vi "WiFi Config.vi"() -> (0 "IP Address":string)   [LabVIEW 2015]
uses:
  <vilib>/LAVA/UI Tools/Engine/Move Speed__lava_lib_ui_tools.ctl
  <vilib>/Utility/miscctls.llb/LVPositionTypeDef.ctl
  Utilities/G1.vi
  <vilib>/Platform/browser.llb/Open URL in Default Browser (string).vi
  <vilib>/MakerHub/Toolbox/LMH-Toolbox.lvlib
panel:
  in  "Overall Help 2":bool
  out "Help 2":string
  out "Tab Control":T1(tab)
  in  "INIT CANCEL":bool
  in  "INIT FRONT":bool
  in  "CON":enum32{"Y", "N"}(radio)
  in  "CON CANCEL":bool
  in  "CON FRONT":bool
  in  "CON BK":bool
  in  "H2 CANCEL":bool
  in  "H1 FRONT":bool
  in  "H1 BK":bool
  in  "H1 CANCEL":bool
  in  "H2 FRONT":bool
  in  "H2 BK":bool
  in  "CONFIG BI WIFI":bool
  in  "CONFIG CUS WIFI":bool
  out "Built-in WiFi":string="172.16.0.1"
  out "USB":string="172.22.11.2"
  in  "H3 CANCEL":bool
  in  "H3 FRONT":bool
  in  "H3 BK":bool
  in  "H4 CANCEL":bool
  in  "H4 FRONT":bool
  in  "H4 BK":bool
  in  "TELL CANCEL":bool
  in  "TELL FRONT":bool
  in  "TELL BK":bool
  in  "TELL CUSTOM IP":string caption="Please enter the IP address"
  in  "Select one":u16(ring)=1 items=["USB", "Built-in WiFi", "Custom WiFi"]
  in  "Finish":bool
  # "Communication Wizard"
  # "Hi! This is your first\nstep in starting the\nrobot. Go ahead!!"
  # "myRIO Connected??\nHave you connected the myRIO\nto your system yet??"
  # "Conecting myRIO: Step 1\nFirst power up myRIO. Wait\nfor a couple of minutes.\nConnect the myRIO via USB or WiFi."
  # "These two should light\nup. \"STATUS\" will turn\noff soon"
  # "Step 2\nOpen the project explorer. Right-click\non myRIO and open properties."
  # "ILLUSTRATION ONLY"
  # "Step 3\nEnter the IP Adddress of myRIO. A\ntable of IP addresses is given below.\nOnce done, click OK."
  # "ILLUSTRATION ONLY"
  # "If you wish to copy the addresses,\ndo it from below"
  # "Step 4\nRight-click on myRIO and\nclick on connect. If you\nget a prompt like the one\nshown in \"Fig 1\" click OK\nor Apply."
  # "ILLUSTRATION ONLY"
  # "Fig 1"
  # "What have you done??\nPlease tell us how have you\nconnected to myRIO. Choose\none option below"
  # "Done!!\nYou are done with connecting with\nmyRIO. Click finish to proceed on to\nthe settings for the robot"
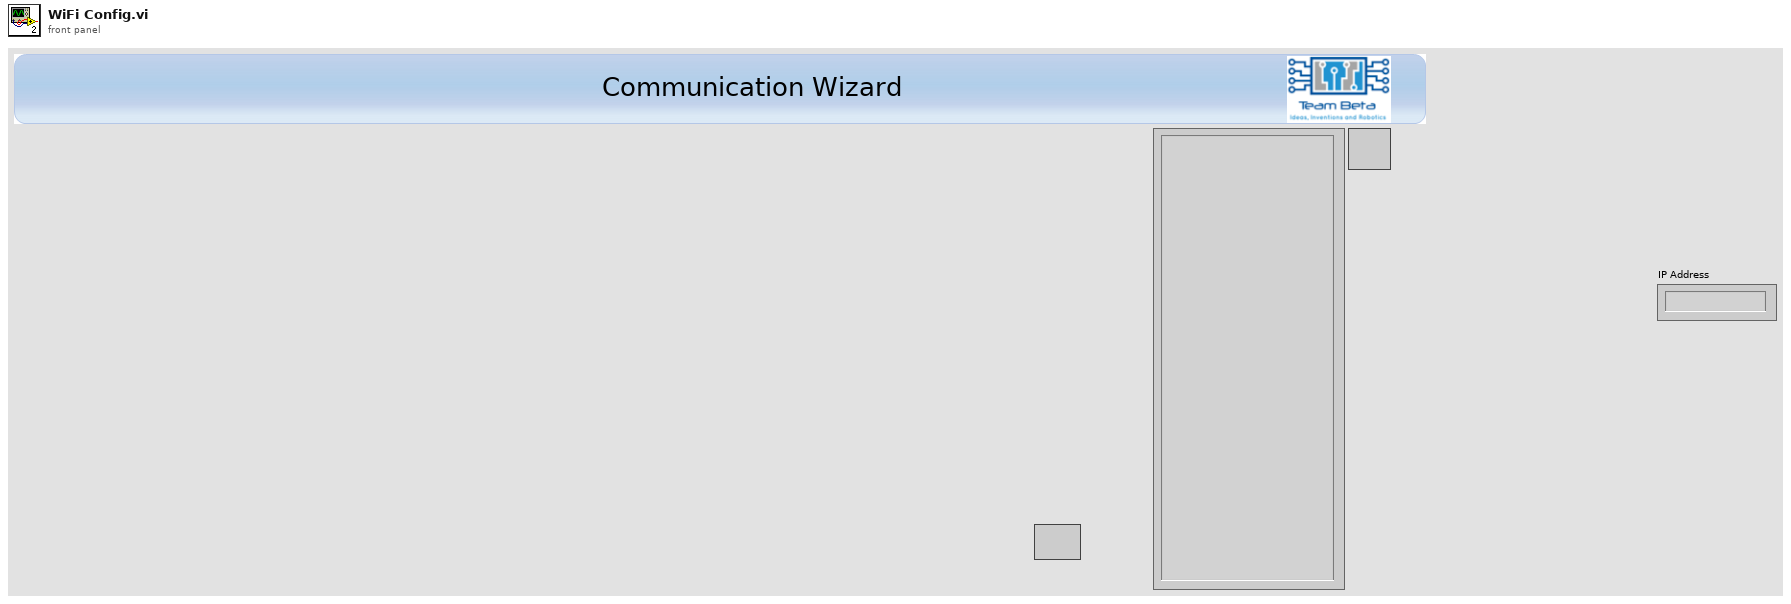
[diagram p1: front panel]
types:
  T1 = enum32{"Init", "myRIO connected?", "H1", "H2", "H3", "H4", "Tell", "Done"}
  T2 = typedef "LVPositionTypeDef.ctl" = cluster{"Left":i32, "Top":i32}
  T3 = typedef "Move Speed__lava_lib_ui_tools.ctl" = enum16{"Normal", "Fast", "Slow", "Instantaneous"}
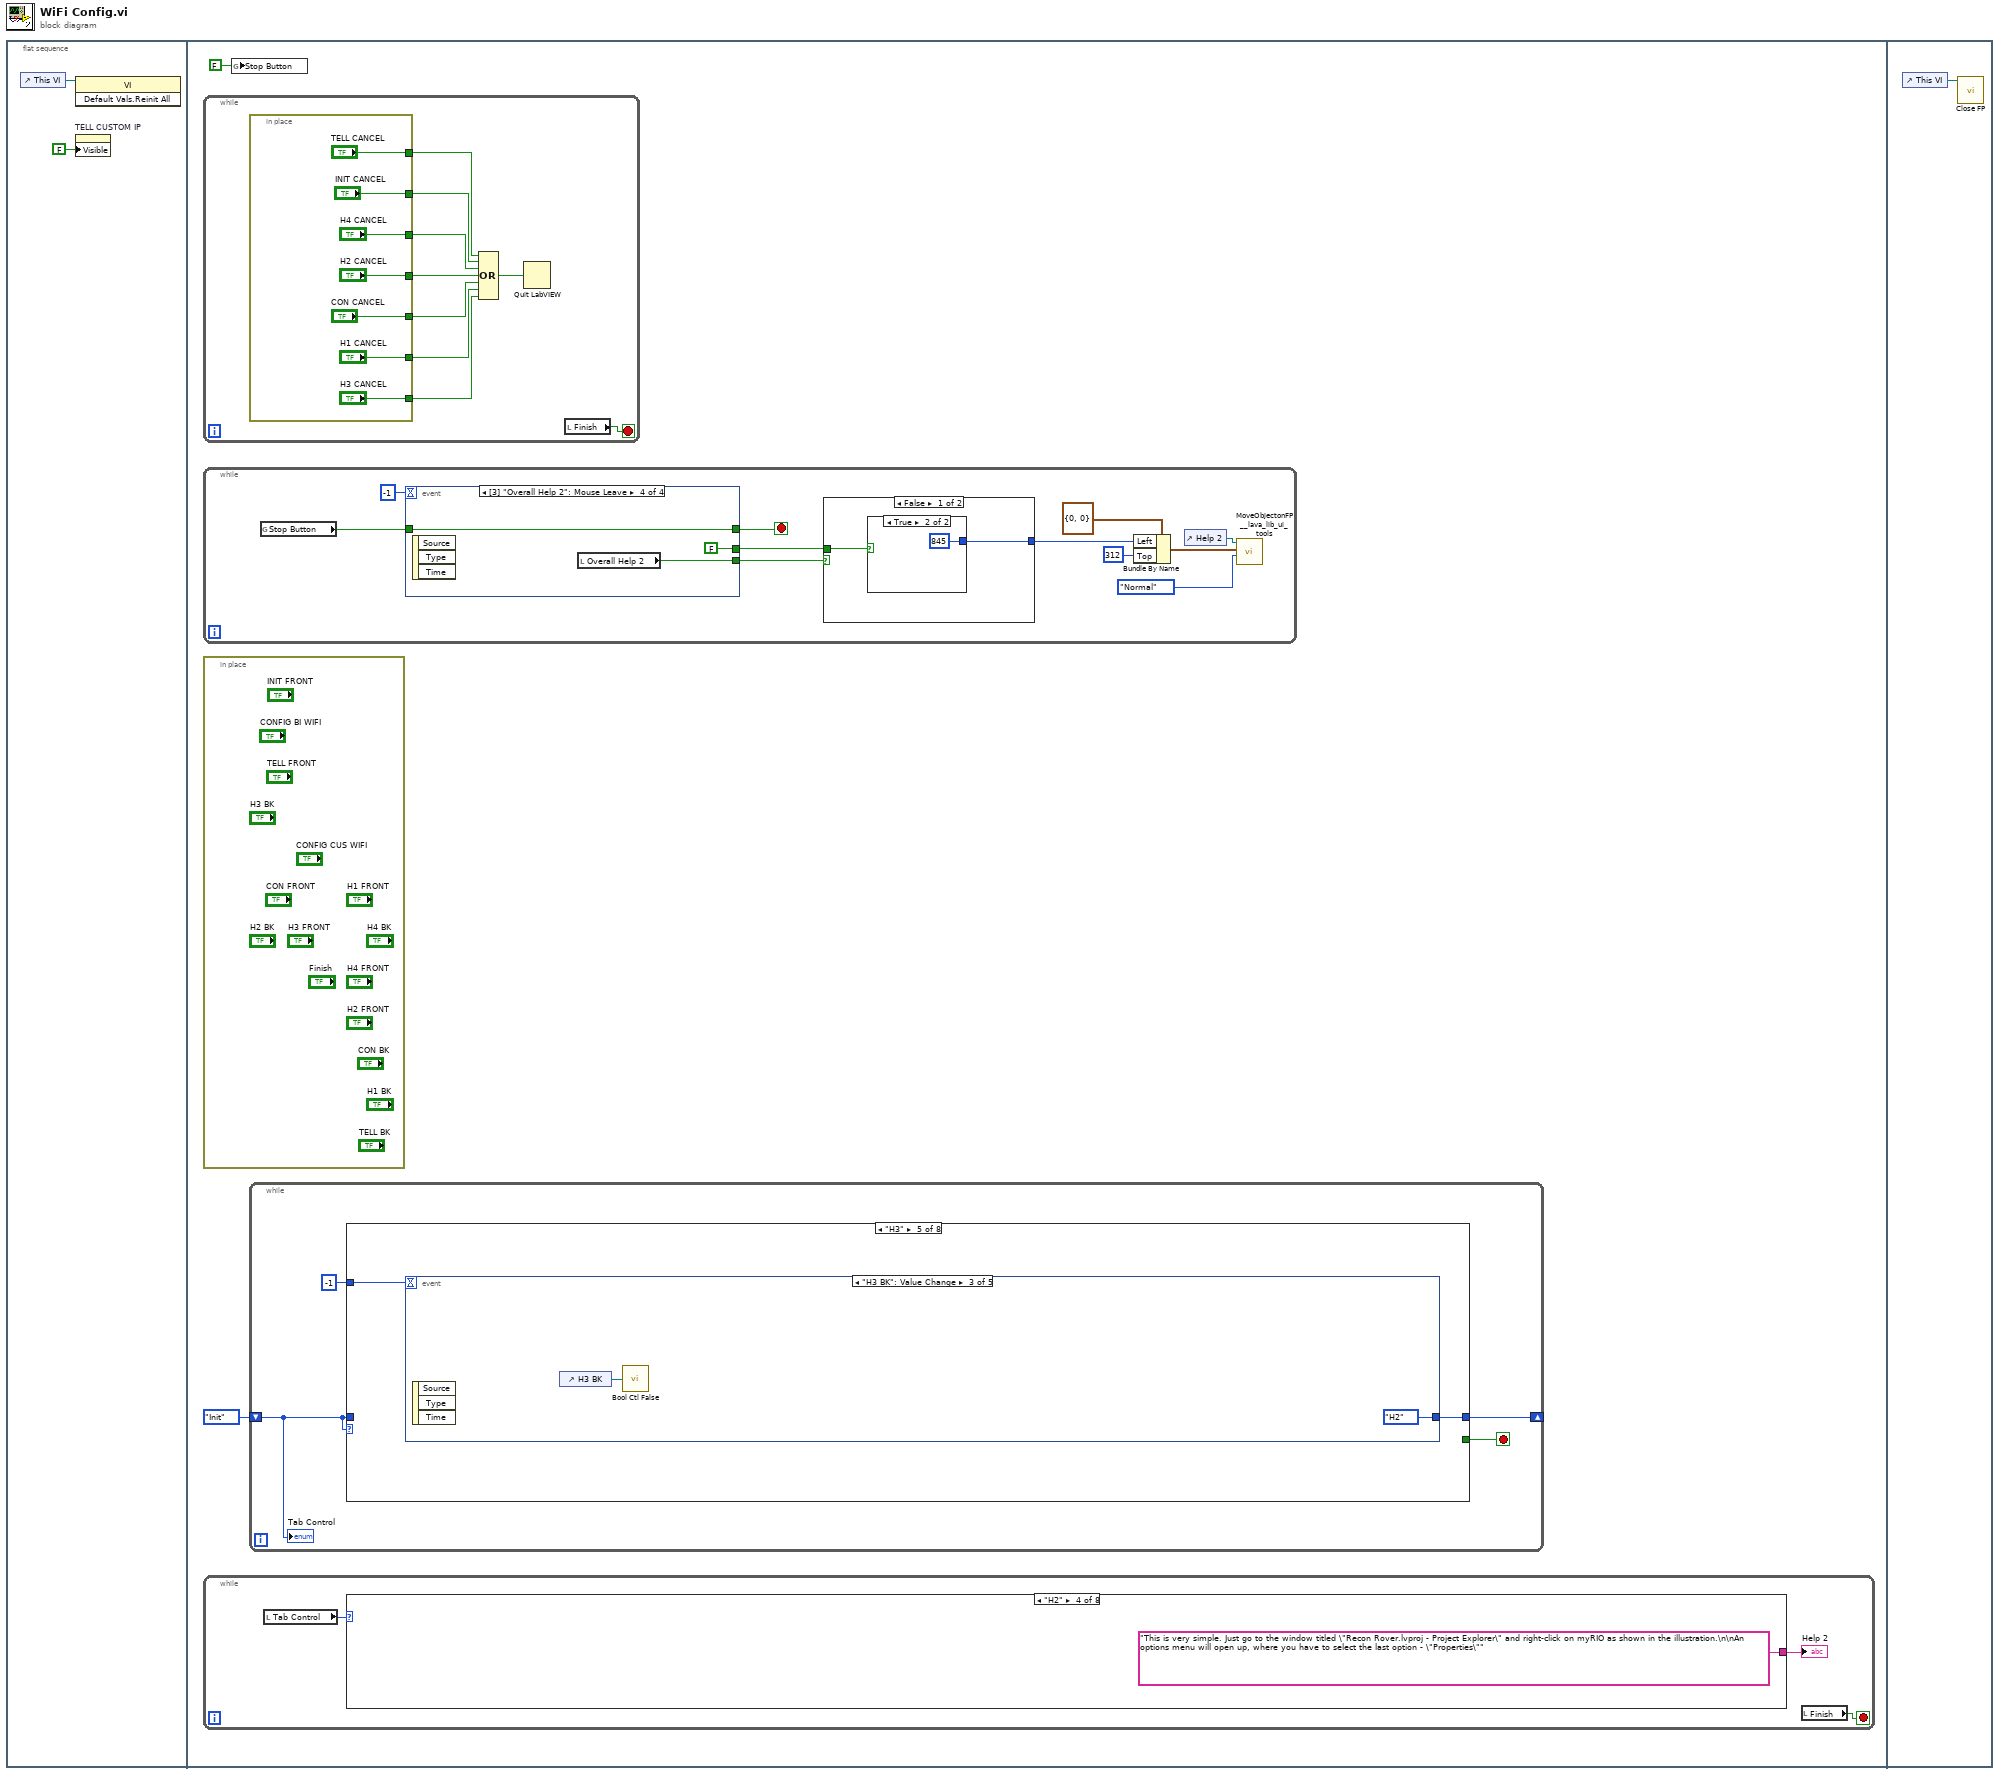
[diagram p0: block diagram]
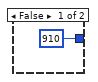
[diagram p2: hidden frame]
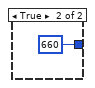
[diagram p3: hidden frame]
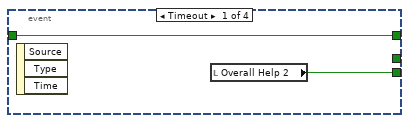
[diagram p4: hidden frame]
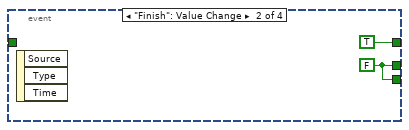
[diagram p5: hidden frame]
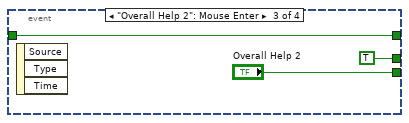
[diagram p6: hidden frame]
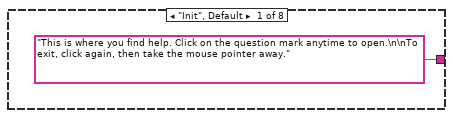
[diagram p7: hidden frame]
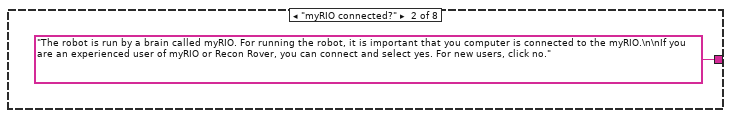
[diagram p8: hidden frame]
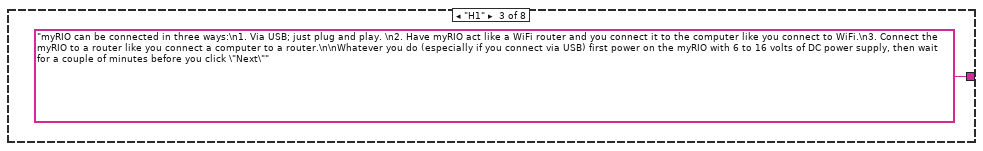
[diagram p9: hidden frame]
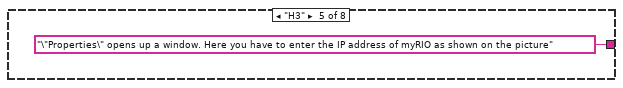
[diagram p10: hidden frame]
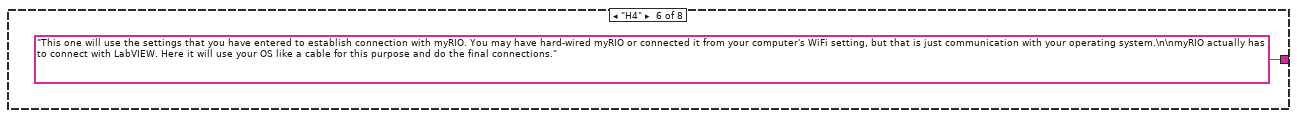
[diagram p11: hidden frame]
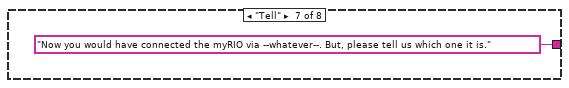
[diagram p12: hidden frame]
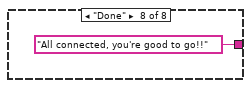
[diagram p13: hidden frame]
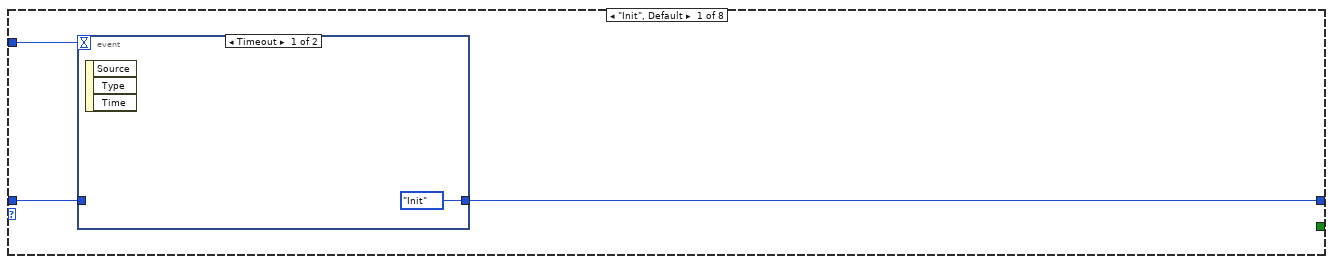
[diagram p14: hidden frame]
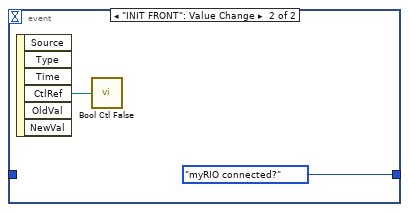
[diagram p15: hidden frame]
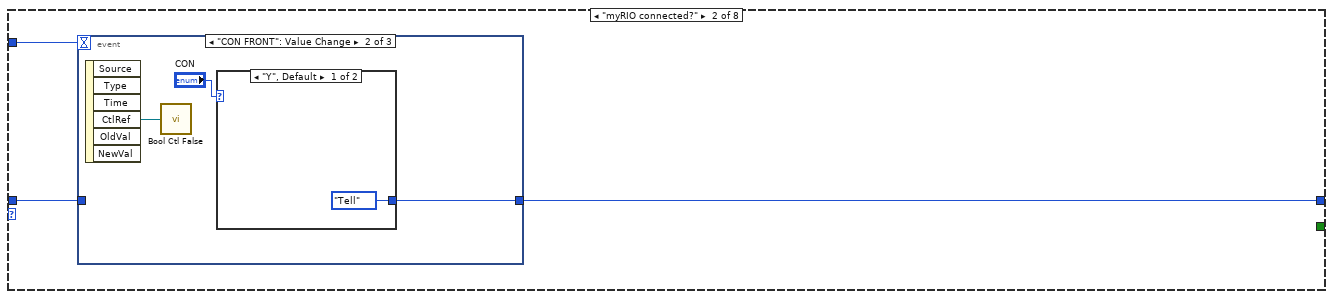
[diagram p16: hidden frame]
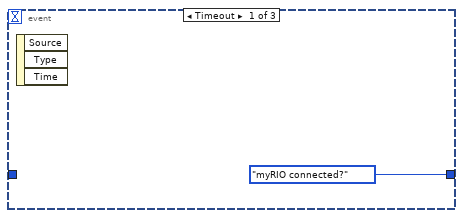
[diagram p17: hidden frame]
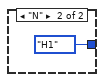
[diagram p18: hidden frame]
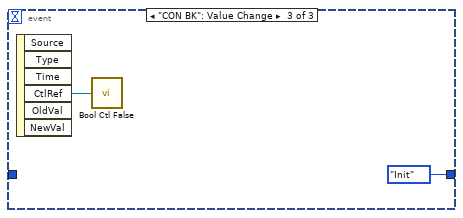
[diagram p19: hidden frame]
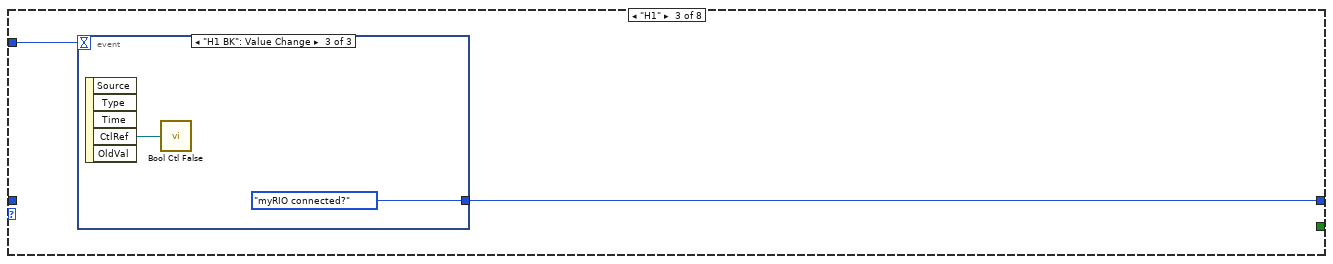
[diagram p20: hidden frame]
diagram:
  n1 = flat-sequence {
    frame #0 {
      n2 = control-ref of="This VI"() -> (w1:refnum<vi>)
      n3 = invoke class="VI" method="Default Vals.Reinit All"(reference=w1) -> ()  [unwired: 2 in, 3 out]
      n4 = property on="TELL CUSTOM IP" class="Str"("Visible"=FALSE) -> ()  [unwired: 2 in, 2 out]
    }
    frame #1 {
      n5 = while {
        stop <- w42 stop-if-true
        n6 = in-place {
          in-place-border: ["TELL CANCEL"] -> w50
          in-place-border: ["INIT CANCEL"] -> w49
          in-place-border: ["H4 CANCEL"] -> w48
          in-place-border: ["H2 CANCEL"] -> w47
          in-place-border: ["CON CANCEL"] -> w46
          in-place-border: ["H1 CANCEL"] -> w45
          in-place-border: ["H3 CANCEL"] -> w44
        }
        n7 = Compound Arithmetic op=OR(w50, w49, w48, w47, w46, w45, w44) -> (w43:bool)
        n8 = Quit LabVIEW(quit? (T)=w43) -> ()
        n9 = local read "Finish"() -> (w42:bool)
      }
      n10 = while {
        stop <- w14 stop-if-true
        n11 = global read "G1.vi" "Stop Button"() -> (w13:bool)
        n12 = event shown="[3] \"Overall Help 2\": Mouse Leave" {
          selector: _ -> [_ _ _ _]
          dyn-events: _ -> [_ _ _ _]
          timeout: -1 -> [_ _ _ _]
          tunnel: [_ w23 TRUE FALSE] -> w10
          tunnel: [w22 w23 "Overall Help 2" w29] -> w9
          tunnel: [w21 TRUE ("Stop Button") w25 w28] -> w14
          tunnel: w13 -> [w21 _ w25 w28]
          event Timeout {
            n13 = event-data() -> ()  [unwired: 1 in, 3 out]
            n14 = local read "Overall Help 2"() -> (w22:bool)
          }
          event "Finish": Value Change {
            w23 = FALSE
            n15 = event-data() -> ()  [unwired: 1 in, 3 out]
          }
          event "Overall Help 2": Mouse Enter {
            n16 = event-data() -> ()  [unwired: 1 in, 3 out]
          }
          event "Overall Help 2": Mouse Leave {
            n17 = event-data() -> ()  [unwired: 1 in, 3 out]
            n18 = local read "Overall Help 2"() -> (w29:bool)
          }
        }
        n19 = case shown="False" w9 {
          tunnel: w10 -> [w17 _]
          tunnel: [w16 660] -> w5
          frame False {
            n20 = case shown="True" w17 {
              tunnel: [910 845] -> w16
              frame False {
              }
              frame True {
              }
            }
          }
          frame True {
          }
        }
        n21 = Bundle By Name(cluster=T2 {"Left"=0, "Top"=0} ("Center Position for Object"), "Left"=w5, "Top"=312) -> (w6:T2)
        n22 = control-ref of="Help 2"() -> (w11:refnum<vi>)
        n23 = call <vilib>:"MoveObjectonFP__lava_lib_ui_tools.vi"("Move Speed (Instantaneous)"=Move_Speed__lava_lib_ui_tools."Normal", "Center Position for Object"=w6, "GObject"=w11) -> ()  [unwired: 7 in, 2 out]
      }
      n24 = in-place {
      }
      n25 = while {
        stop <- w33 stop-if-true
        n26 = local read "Tab Control"() -> (w32:T1)
        n27 = case shown="\"H2\"" w32 {
          tunnel: ["This is where you find help. Click on the question mark anytime to open.\n\nTo exit, click again, then take the mouse pointer away." "The robot is run by a brain called myRIO. For running the robot, it is important that you computer is connected to the myRIO.\n\nIf you are an experienced user of myRIO or Recon Rover, you can connect and select yes. For new users, click no." "myRIO can be connected in three ways:\n1. Via USB; just plug and play. \n2. Have myRIO act like a WiFi router and you connect it to the computer like you connect to WiFi.\n3. Connect the myRIO to a router like you connect a computer to a router.\n\nWhatever you do (especially if you connect via USB) first power on the myRIO with 6 to 16 volts of DC power supply, then wait for a couple of minutes before you click \"Next\"" "This is very simple. Just go to the window titled \"Recon Rover.lvproj - Project Explorer\" and right-click on myRIO as shown in the illustration.\n\nAn options menu will open up, where you have to select the last option - \"Properties\"" "\"Properties\" opens up a window. Here you have to enter the IP address of myRIO as shown on the picture" "This one will use the settings that you have entered to establish connection with myRIO. You may have hard-wired myRIO or connected it from your computer's WiFi setting, but that is just communication with your operating system.\n\nmyRIO actually has to connect with LabVIEW. Here it will use your OS like a cable for this purpose and do the final connections." "Now you would have connected the myRIO via --whatever--. But, please tell us which one it is." "All connected, you're good to go!!"] -> w31
          frame "Init", Default {
          }
          frame "myRIO connected?" {
          }
          frame "H1" {
          }
          frame "H2" {
          }
          frame "H3" {
          }
          frame "H4" {
          }
          frame "Tell" {
          }
          frame "Done" {
          }
        }
        "Help 2" <- w31
        n28 = local read "Finish"() -> (w33:bool)
      }
      n29 = global write "G1.vi" "Stop Button"(FALSE ("Stop Button")) -> ()
      n30 = while {
        shift-right: [w61] -> _
        shift-left: T1."Init" ("Tab Control 2") -> [w60]
        stop <- w58 stop-if-true
        n31 = case shown="\"H3\"" w60 {
          tunnel: [w64 w68 w79 w86 w94 w108 w115 w137] -> w61
          tunnel: w60 -> [w63 w70 _ _ _ _ _ _]
          tunnel: -1 -> [w62 w69 w80 w87 w93 w109 w116 w138]
          tunnel: [_ _ _ _ _ _ _ w136] -> w58
          frame "Init", Default {
            n32 = event shown="[0] Timeout" {
              selector: _ -> [_ _]
              dyn-events: _ -> [_ _]
              timeout: w62 -> [_ _]
              tunnel: [T1."Init" ("Tab Control 2") T1."myRIO connected?" ("Tab Control 2")] -> w64
              tunnel: w63 -> [_ _]
              event Timeout {
                n33 = event-data() -> ()  [unwired: 1 in, 3 out]
              }
              event "INIT FRONT": Value Change {
                n34 = event-data() -> ("CtlRef"=w66:refnum<vi>)  [unwired: 1 in, 5 out]
                n35 = call "Bool Ctl False.vi"("Control Ref"=w66) -> ()
              }
            }
          }
          frame "myRIO connected?" {
            n36 = event shown="[1] \"CON FRONT\": Value Change" {
              selector: _ -> [_ _ _]
              dyn-events: _ -> [_ _ _]
              timeout: w69 -> [_ _ _]
              tunnel: w70 -> [_ _ _]
              tunnel: [T1."myRIO connected?" ("Tab Control 2") w73 T1."Init" ("Tab Control 2")] -> w68
              event Timeout {
                n37 = event-data() -> ()  [unwired: 1 in, 3 out]
              }
              event "CON FRONT": Value Change {
                n38 = event-data() -> ("CtlRef"=w72:refnum<vi>)  [unwired: 1 in, 5 out]
                n39 = call "Bool Ctl False.vi"("Control Ref"=w72) -> ()
                n40 = case shown="\"Y\", Default" "CON" {
                  tunnel: [T1."Tell" ("Tab Control 2") T1."H1" ("Tab Control 2")] -> w73
                  frame "Y", Default {
                  }
                  frame "N" {
                  }
                }
              }
              event "CON BK": Value Change {
                n41 = event-data() -> ("CtlRef"=w77:refnum<vi>)  [unwired: 1 in, 5 out]
                n42 = call "Bool Ctl False.vi"("Control Ref"=w77) -> ()
              }
            }
          }
          frame "H1" {
            n43 = event shown="[2] \"H1 BK\": Value Change" {
              selector: _ -> [_ _ _]
              dyn-events: _ -> [_ _ _]
              timeout: w80 -> [_ _ _]
              tunnel: [T1."H1" ("Tab Control 2") T1."H2" ("Tab Control 2") T1."myRIO connected?" ("Tab Control 2")] -> w79
              event Timeout {
                n44 = event-data() -> ()  [unwired: 1 in, 3 out]
              }
              event "H1 FRONT": Value Change {
                n45 = event-data() -> ("CtlRef"=w82:refnum<vi>)  [unwired: 1 in, 4 out]
                n46 = call "Bool Ctl False.vi"("Control Ref"=w82) -> ()
              }
              event "H1 BK": Value Change {
                n47 = event-data() -> ("CtlRef"=w84:refnum<vi>)  [unwired: 1 in, 4 out]
                n48 = call "Bool Ctl False.vi"("Control Ref"=w84) -> ()
              }
            }
          }
          frame "H2" {
            n49 = event shown="[1] \"H2 FRONT\": Value Change" {
              selector: _ -> [_ _ _]
              dyn-events: _ -> [_ _ _]
              timeout: w87 -> [_ _ _]
              tunnel: [T1."H2" ("Tab Control 2") T1."H3" ("Tab Control 2") T1."H1" ("Tab Control 2")] -> w86
              event Timeout {
                n50 = event-data() -> ()  [unwired: 1 in, 3 out]
              }
              event "H2 FRONT": Value Change {
                n51 = event-data() -> ("CtlRef"=w89:refnum<vi>)  [unwired: 1 in, 5 out]
                n52 = call "Bool Ctl False.vi"("Control Ref"=w89) -> ()
              }
              event "H2 BK": Value Change {
                n53 = event-data() -> ("CtlRef"=w92:refnum<vi>)  [unwired: 1 in, 5 out]
                n54 = call "Bool Ctl False.vi"("Control Ref"=w92) -> ()
              }
            }
          }
          frame "H3" {
            n55 = event shown="[2] \"H3 BK\": Value Change" {
              selector: _ -> [_ _ _ _ _]
              dyn-events: _ -> [_ _ _ _ _]
              timeout: w93 -> [_ _ _ _ _]
              tunnel: [T1."H3" ("Tab Control 2") T1."H4" ("Tab Control 2") T1."H2" ("Tab Control 2") T1."H3" ("Tab Control 2") T1."H3" ("Tab Control 2")] -> w94
              event Timeout {
                n56 = event-data() -> ()  [unwired: 1 in, 3 out]
                "USB" <- "172.22.11.2" ("USB")
                "Built-in WiFi" <- "172.16.0.1" ("Built-in WiFi")
              }
              event "H3 FRONT": Value Change {
                n57 = event-data() -> ()  [unwired: 1 in, 3 out]
                n58 = control-ref of="H3 FRONT"() -> (w98:refnum<vi>)
                n59 = call "Bool Ctl False.vi"("Control Ref"=w98) -> ()
              }
              event "H3 BK": Value Change {
                n60 = event-data() -> ()  [unwired: 1 in, 3 out]
                n61 = control-ref of="H3 BK"() -> (w100:refnum<vi>)
                n62 = call "Bool Ctl False.vi"("Control Ref"=w100) -> ()
              }
              event "CONFIG CUS WIFI": Value Change {
                n63 = event-data() -> ()  [unwired: 1 in, 3 out]
                n64 = control-ref of="CONFIG CUS WIFI"() -> (w104:refnum<vi>)
                n65 = call "Bool Ctl False.vi"("Control Ref"=w104) -> ()
                n66 = call-poly <vilib>:"Open URL in Default Browser.vi"("URL"="file:///C:/Program%20Files%20(x86)/National%20Instruments/LabVIEW%202015/resource/myRIO/Tutorials/ConfigureWifi/configurewifi2.html") -> ()  [unwired: 5 in, 2 out]
              }
              event "CONFIG BI WIFI": Value Change {
                n67 = event-data() -> ()  [unwired: 1 in, 3 out]
                n68 = control-ref of="CONFIG BI WIFI"() -> (w105:refnum<vi>)
                n69 = call "Bool Ctl False.vi"("Control Ref"=w105) -> ()
                n70 = call-poly <vilib>:"Open URL in Default Browser.vi"("URL"="file:///C:/Program%20Files%20(x86)/National%20Instruments/LabVIEW%202015/resource/myRIO/Tutorials/ConfigureWifi/configurewifi1.html") -> ()  [unwired: 5 in, 2 out]
              }
            }
          }
          frame "H4" {
            n71 = event shown="[2] \"H4 BK\": Value Change" {
              selector: _ -> [_ _ _]
              dyn-events: _ -> [_ _ _]
              timeout: w109 -> [_ _ _]
              tunnel: [T1."H4" ("Tab Control 2") T1."Tell" ("Tab Control 2") T1."H3" ("Tab Control 2")] -> w108
              event Timeout {
                n72 = event-data() -> ()  [unwired: 1 in, 3 out]
              }
              event "H4 FRONT": Value Change {
                n73 = event-data() -> ("CtlRef"=w112:refnum<vi>)  [unwired: 1 in, 5 out]
                n74 = call "Bool Ctl False.vi"("Control Ref"=w112) -> ()
              }
              event "H4 BK": Value Change {
                n75 = event-data() -> ("CtlRef"=w114:refnum<vi>)  [unwired: 1 in, 5 out]
                n76 = call "Bool Ctl False.vi"("Control Ref"=w114) -> ()
              }
            }
          }
          frame "Tell" {
            n77 = event shown="[0] Timeout" {
              selector: _ -> [_ _ _ _]
              dyn-events: _ -> [_ _ _ _]
              timeout: w116 -> [_ _ _ _]
              tunnel: [T1."Tell" ("Tab Control 2") T1."Done" ("Tab Control 2") T1."Tell" ("Tab Control 2") w131] -> w115
              event Timeout {
                n78 = event-data() -> ()  [unwired: 1 in, 3 out]
              }
              event "TELL FRONT": Value Change {
                n79 = event-data() -> ("CtlRef"=w122:refnum<vi>)  [unwired: 1 in, 4 out]
                n80 = call "Bool Ctl False.vi"("Control Ref"=w122) -> ()
                n81 = case shown="1" "Select one" {
                  tunnel: ["172.22.11.2" ("TELL CUSTOM IP") "172.16.0.1" ("TELL CUSTOM IP") w125] -> w120
                  tunnel: "TELL CUSTOM IP" -> [_ _ w125]
                  frame 0, Default {
                  }
                  frame 1 {
                  }
                  frame 2 {
                  }
                }
                "IP Address" <- w120
              }
              event "Select one": Value Change {
                n82 = event-data() -> ("CtlRef"=w128:refnum<vi>)  [unwired: 1 in, 5 out]
                n83 = property class="Ring (strict)"(reference=w128) -> ("Value"=w127:u16)  [unwired: 1 in, 2 out]
                n84 = Equal?(x=w127, y=u16 2) -> (x = y?=w129:bool)
                n85 = property on="TELL CUSTOM IP" class="Str"("Visible"=w129) -> ()  [unwired: 2 in, 2 out]
              }
              event "TELL BK": Value Change {
                n86 = event-data() -> ("CtlRef"=w133:refnum<vi>)  [unwired: 1 in, 4 out]
                n87 = call "Bool Ctl False.vi"("Control Ref"=w133) -> ()
                n88 = local read "CON"() -> (w132:enum32{"Y", "N"})
                n89 = case shown="\"Y\", Default" w132 {
                  tunnel: [T1."myRIO connected?" ("Tab Control 2") T1."H4" ("Tab Control 2")] -> w131
                  frame "Y", Default {
                  }
                  frame "N" {
                  }
                }
              }
            }
          }
          frame "Done" {
            n90 = event shown="[1] \"Finish\": Value Change" {
              selector: _ -> [_ _]
              dyn-events: _ -> [_ _]
              timeout: w138 -> [_ _]
              tunnel: [T1."Done" ("Tab Control 2") T1."Done" ("Tab Control 2")] -> w137
              tunnel: [_ TRUE] -> w136
              event Timeout {
                n91 = event-data() -> ()  [unwired: 1 in, 3 out]
              }
              event "Finish": Value Change {
                n92 = event-data() -> ()  [unwired: 1 in, 3 out]
                n93 = control-ref of="Finish"() -> (w142:refnum<vi>)
                n94 = call "Bool Ctl False.vi"("Control Ref"=w142) -> ()
              }
            }
          }
        }
        "Tab Control" <- w60
      }
    }
    frame #2 {
      n95 = control-ref of="This VI"() -> (w143:refnum<vi>)
      n96 = call <vilib>:"Close FP.vi"("VI Ref"=w143) -> ()  [unwired: 10 in, 1 out]
    }
  }
